vi "Remove Quotes if Existing.vi"(1 "String":string) -> (0 "String out":string)   [LabVIEW 2015, in "YAML Parser.lvclass"]
uses:
  YAML Parser.lvclass
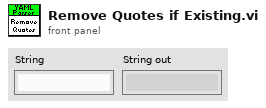
[diagram p1: front panel]
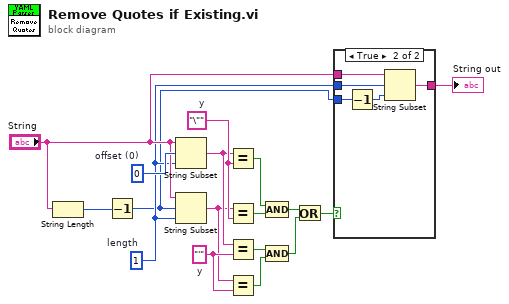
[diagram p0: block diagram]
diagram:
  w6 = "'"  # y
  w13 = "\""  # y
  w10 = 1  # length
  w17 = 0  # offset (0)
  n1 = String Length(string="String") -> (length=w16:i32)
  n2 = Decrement(x=w16) -> (x-1=w9:i32)
  n3 = String Subset(string="String", offset (0)=w17, length (rest)=w10) -> (substring=w7:string)
  n4 = String Subset(string="String", offset (0)=w9, length (rest)=w10) -> (substring=w5:string)
  n5 = Equal?(x=w7, y=w13) -> (x = y?=w15:bool)
  n6 = Equal?(x=w5, y=w13) -> (x = y?=w14:bool)
  n7 = Equal?(x=w7, y=w6) -> (x = y?=w4:bool)
  n8 = Equal?(x=w5, y=w6) -> (x = y?=w3:bool)
  n9 = Compound Arithmetic op=AND(w15, w14) -> (w8:bool)
  n10 = Compound Arithmetic op=AND(w4, w3) -> (w2:bool)
  n11 = Or(x=w8, y=w2) -> (x .or. y?=w1:bool)
  n12 = case shown="True" w1 {
    tunnel: [w18 w22] -> w12
    tunnel: "String" -> [w18 w23]
    tunnel: w10 -> [_ w21]
    tunnel: w9 -> [_ w20]
    frame False {
    }
    frame True {
      n13 = Decrement(x=w20) -> (x-1=w19:i32)
      n14 = String Subset(string=w23, offset (0)=w21, length (rest)=w19) -> (substring=w22:string)
    }
  }
  "String out" <- w12
